vi "基本信息解析.vi"(10 "线号":i32, 11 "基本信息":T1={"序号"=12.0, "线总数"=1.0, "布线板长"=450.0, "布线板宽"=200.0, "Mark1X"=12500.0, "Mark1Y"=12500.0, "Mark2X"=437500.0, "Mark2Y"=187500.0, "1阶段线数"=[], "2阶段线数"=[], "3阶段线数"=[]}) -> (3 "添加的数组":dbl[](array[numeric]))   [LabVIEW 2014]
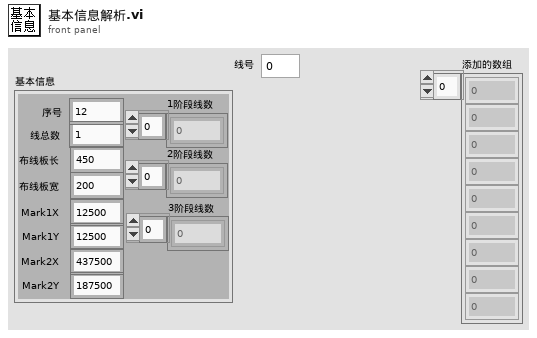
[diagram p1: front panel]
types:
  T1 = typedef "基本信息.ctl" = cluster{"序号":dbl, "线总数":dbl, "布线板长":dbl, "布线板宽":dbl, "Mark1X":dbl, "Mark1Y":dbl, "Mark2X":dbl, "Mark2Y":dbl, "1阶段线数":dbl[], "2阶段线数":dbl[], "3阶段线数":dbl[]}
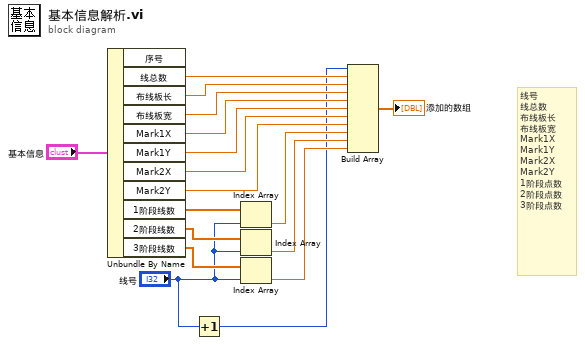
[diagram p0: block diagram]
diagram:
  # "线号\n线总数\n布线板长\n布线板宽\nMark1X\nMark1Y\nMark2X\nMark2Y\n1阶段点数\n2阶段点数\n3阶段点数"
  n1 = Unbundle By Name("基本信息") -> ("线总数"=w16:dbl, "布线板长"=w15:dbl, "布线板宽"=w14:dbl, "Mark1X"=w13:dbl, "Mark1Y"=w12:dbl, "Mark2X"=w11:dbl, "Mark2Y"=w10:dbl, "1阶段线数"=w9:dbl[], "2阶段线数"=w7:dbl[], "3阶段线数"=w6:dbl[])  [unwired: 1 out]
  n2 = Increment(x="线号") -> (x+1=w1:i32)
  n3 = Index Array(array=w9, index="线号") -> (element=w8:dbl)
  n4 = Index Array(array=w7, index="线号") -> (element=w5:dbl)
  n5 = Index Array(array=w6, index="线号") -> (element=w4:dbl)
  n6 = Build Array(w1, w16, w15, w14, w13, w12, w11, w10, w8, w5, w4) -> (→"添加的数组":dbl[])
